vi "Ctor.vi"(8 "error in (no error)":errorcluster, 11 "DeviceListPanel in":refnum<class "DeviceListPanel.lvclass">) -> (0 "error out":errorcluster, 3 "DeviceListPanel out":refnum<class "DeviceListPanel.lvclass">)   [LabVIEW 2020, in "PicoG-App.lvlib" / "DeviceListPanel.lvclass"]
uses:
  DeviceListPanel.lvclass
  Device/Device Key.ctl
  Device and Panel.ctl
  Device/Device.lvclass
  DeviceArrayPanel/DeviceArrayPanel.lvclass
  Ref Data.ctl
  DeviceListPanel.lvclass/DeviceListPanel.ctl
  9e649c8e-63a0-4e9d-aad4-ed1dc7d5ad5e.vi
  <vilib>/IlluminatedG/IG OOPanel/OOPanel/Panel/Panel.lvclass
  <vilib>/IlluminatedG/IG OOPanel/OOPanel/ArrayManager/ArrayManager.lvclass
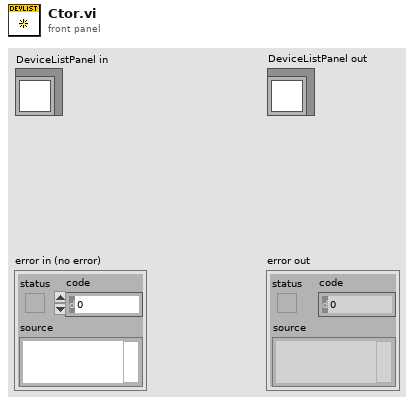
[diagram p1: front panel]
types:
  T1 = typedef "PicoG-App.lvlib/DeviceListPanel.lvclass/Ref Data.ctl" = cluster{"Map":map{T2, T3}}
  T2 = typedef "PicoG-App.lvlib/Device.lvclass/Device Key.ctl" = cluster{"Platform":string, "Board":string, "ID":string}
  T3 = typedef "PicoG-App.lvlib/DeviceListPanel.lvclass/Device and Panel.ctl" = cluster{"Device":refnum<class "Device.lvclass">, "Panel":refnum<class "DeviceArrayPanel.lvclass">}
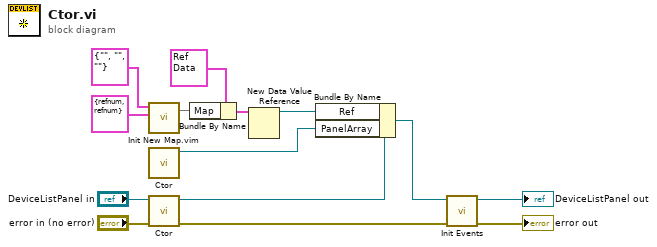
[diagram p0: block diagram]
diagram:
  n1 = call "Init New Map.vim"("Value Type"=T3 {"Device"=refnum, "Panel"=refnum} ("Device and Panel"), "Key Type"=T2 {"Platform"="", "Board"="", "ID"=""} ("Device Key")) -> ("Map"=w3:map{T2, T3})  [unwired: 5 in]
  n2 = call <vilib>:"Ctor.vi"() -> ("PanelArray"=w1:refnum<class "ArrayManager.lvclass">)  [unwired: 10 in, 1 out]
  n3 = call-parent <vilib>:"Ctor.vi"("error in (no error)"="error in (no error)", "Panel in"="DeviceListPanel in") -> ("error out"=w11:errorcluster, "Panel out"=w12:refnum<class "DeviceListPanel.lvclass">)  [unwired: 8 in]
  n4 = Bundle By Name(cluster=T1 {"Map"={}} ("Ref Data"), "Map"=w3) -> (w4:T1)
  n5 = New Data Value Reference(data value=w4) -> (data value reference=w2:refnum<data-value>)  [unwired: 1 in, 1 out]
  n6 = Bundle By Name(cluster=w12, "Ref"=w2, "PanelArray"=w1) -> (w5:refnum<class "DeviceListPanel.lvclass">)
  n7 = call "Init Events.vi"("error in (no error)"=w11, "DeviceListPanel in"=w5) -> ("error out"=→"error out":errorcluster, "DeviceListPanel out"=→"DeviceListPanel out":refnum<class "DeviceListPanel.lvclass">)  [unwired: 8 in]
